vi "Set Measured Flow Rate as Zero.vi"(8 "error in (no error)":errorcluster, 11 "RRG in":refnum<class "Eltochpribor RRG.lvclass">) -> (0 "error out":errorcluster, 3 "RRG out":refnum<class "Eltochpribor RRG.lvclass">)   [LabVIEW 2015, in "Eltochpribor RRG.lvclass"]
doc: "Sets current measured flow rate as zero."
uses:
  Eltochpribor RRG.lvclass
  Modbus Client/PL Modbus Client.lvclass
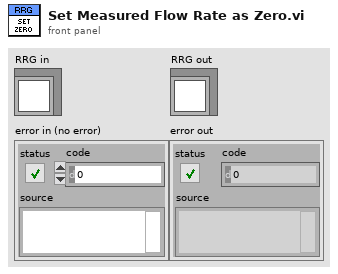
[diagram p1: front panel]
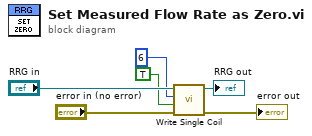
[diagram p0: block diagram]
diagram:
  n1 = call "Write Single Coil.vi"("error in (no error)"="error in (no error)", "value"=TRUE, "address"=u16 6, "MODBUS in"="RRG in") -> ("error out"=→"error out":errorcluster, "MODBUS out"=→"RRG out":refnum<class "Eltochpribor RRG.lvclass">)  [unwired: 6 in]
